vi "Benchmark (SubVI).vi"(10 "Tag Lookup":enum32{"By Name", "By Ref"}(radio)=enum."By Ref", 11 "#Tags":i32=100000) -> (0 "Values":dbl[](array[numeric]), 1 "Read Time":dbl format="%#_g s", 2 "Write Time":dbl format="%#_g s", 3 "Creation Time":dbl format="%#_g s")   [LabVIEW 2018]
doc: "_Test_"
uses:
  Tag/Tag.lvclass/Tag.ctl
  Core/Tag Core.lvclass/Tag Core.ctl
  9bdda2ff-a9dc-4140-9278-b7922a7097c1.vi
  2d795fc3-3ce1-4465-af3b-7f0aa2d422e4.vi
  f807e1ac-a0a3-4e29-b252-0f3a40794f64.vi
  62b6eeaa-51de-4935-a683-d32b75056f49.vi
  45d263af-4112-4fe1-aae2-d3d76b89cb2f.vi
  Tag/Construct.vi
  2d795fc3-3ce1-4465-af3b-7f0aa2d422e4.vi/dad9aa0d-4427-44e9-8a16-aab4251f8442.vi
  2d795fc3-3ce1-4465-af3b-7f0aa2d422e4.vi/85ef243b-a7be-4ddd-aba5-de1810920a44.vi
  f807e1ac-a0a3-4e29-b252-0f3a40794f64.vi/b0e6ee81-700c-4175-ad68-c0a6ecad06c4.vi
  Core/Get Tag.vi
  f807e1ac-a0a3-4e29-b252-0f3a40794f64.vi/af024140-0f6e-4ec8-bc40-cd99cce420e6.vi
  62b6eeaa-51de-4935-a683-d32b75056f49.vi/23fa4edd-30cd-4554-957f-93b0c616928a.vi
  62b6eeaa-51de-4935-a683-d32b75056f49.vi/45e37831-75fa-4a91-aa24-5e089f5f592b.vi
  45d263af-4112-4fe1-aae2-d3d76b89cb2f.vi/a499805a-9911-40c2-9faf-cbd2dbdf1bc0.vi
  45d263af-4112-4fe1-aae2-d3d76b89cb2f.vi/4da4ad56-3947-4053-a029-ec9f142512c4.vi
  Tag/Write Value with Timestamp.vi
  Tag/Read Value.vi
  Tag/Read Timestamp.vi
  Tools/Variant to DBL.vi
  Tag/Set Properties from Initial.vi
  Core/Add Tag.vi
  Core/Get Tag LUT.vi
  <vilib>/Utility/error.llb/Error Cluster From Error Code.vi
  <vilib>/Utility/Data Type/Get Type Information.vi
  Tag/Tag.lvclass
  Core/Tag Core.lvclass
panel:
  out "Read Time / Tag":dbl format="%#_g s"
  out "Write Time / Tag":dbl format="%#_g s"
  out "Creation Time / Tag":dbl format="%#_g s"
  # "Totals"
  # "Per Tag"
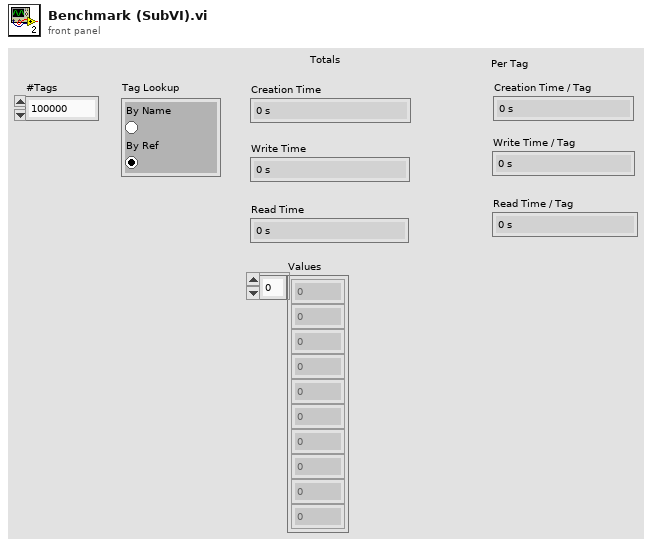
[diagram p1: front panel]
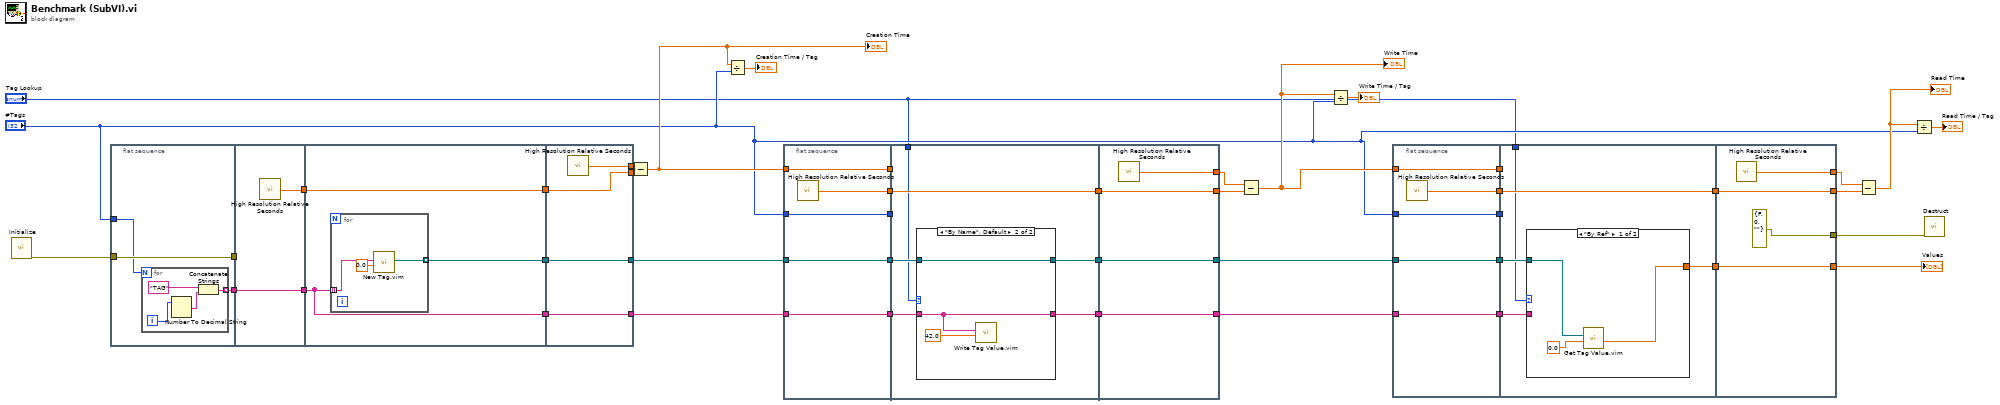
[diagram p0: block diagram]
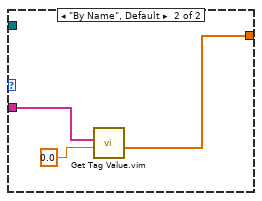
[diagram p2: hidden frame]
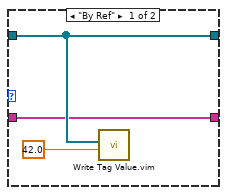
[diagram p3: hidden frame]
diagram:
  n1 = call "Initialize.vi"() -> ("error out"=w39:errorcluster)  [unwired: 11 in]
  n2 = flat-sequence {
    tunnel: w39 -> [w46]
    tunnel: "#Tags" -> [w45]
    tunnel: [w46] -> w23
    tunnel: [w44] -> w21
    tunnel: [w52] -> w42
    tunnel: w23 -> [_]
    tunnel: [w51] -> w22
    tunnel: w21 -> [w51]
    tunnel: [w55] -> w43
    tunnel: w42 -> [w55]
    tunnel: w22 -> [w54]
    tunnel: [w54] -> w18
    tunnel: [w53] -> w7
    tunnel: w43 -> [w61]
    tunnel: [w62] -> w41
    tunnel: [w61] -> w40
    tunnel: [w60] -> w19
    tunnel: w18 -> [w60]
    tunnel: [w59] -> w5
    tunnel: w7 -> [w59]
    frame #0 {
      n3 = for {
        N: w45 -> [_]
        tunnel: [w47] -> w44 mode=indexing
        i -> [w48]
        n4 = Number To Decimal String(number=w48) -> (decimal integer string=w50:string)  [unwired: 1 in]
        n5 = Concatenate Strings("TAG", w50) -> (w47:string)
      }
    }
    frame #1 {
      n6 = call <vilib>:"High Resolution Relative Seconds.vi"() -> ("relative seconds"=w52:dbl)
    }
    frame #2 {
      n7 = for {
        tunnel: w54 -> [w57] mode=indexing
        tunnel: [w56] -> w53 mode=indexing
        n8 = call "New Tag.vim"("Initial Value"=0.0, "Tag Name"=w57) -> ("Tag Ref out"=w56:refnum<data-value>)  [unwired: 8 in, 1 out]
      }
    }
    frame #3 {
      n9 = call <vilib>:"High Resolution Relative Seconds.vi"() -> ("relative seconds"=w62:dbl)
    }
  }
  n10 = Subtract(x=w41, y=w40) -> (x-y=w14:dbl)
  "Creation Time" <- w14
  n11 = Divide(x=w14, y="#Tags") -> (x/y=→"Creation Time / Tag":dbl)
  n12 = flat-sequence {
    tunnel: w14 -> [w67]
    tunnel: [w67] -> w38
    tunnel: [w66] -> w36
    tunnel: [w65] -> w35
    tunnel: "#Tags" -> [w65]
    tunnel: [w64] -> w20
    tunnel: w19 -> [w64]
    tunnel: [w63] -> w6
    tunnel: w5 -> [w63]
    tunnel: w38 -> [_]
    tunnel: [w73] -> w37
    tunnel: w36 -> [w73]
    tunnel: w35 -> [_]
    tunnel: w20 -> [w70]
    tunnel: [w69] -> w15
    tunnel: w6 -> [w72]
    tunnel: [w68] -> w2
    tunnel: "Tag Lookup" -> [w71]
    tunnel: w37 -> [w83]
    tunnel: [w83] -> w33
    tunnel: [w82] -> w34
    tunnel: [w81] -> w16
    tunnel: w15 -> [w81]
    tunnel: [w80] -> w3
    tunnel: w2 -> [w80]
    frame #0 {
      n13 = call <vilib>:"High Resolution Relative Seconds.vi"() -> ("relative seconds"=w66:dbl)
    }
    frame #1 {
      n14 = case shown="\"By Name\", Default" w71 {
        tunnel: w72 -> [w75 w77]
        tunnel: w70 -> [w74 w78]
        tunnel: [w74 w78] -> w69
        tunnel: [w75 w77] -> w68
        frame "By Ref" {
          n15 = call "Write Tag Value.vim"("Value"=42.0, "Tag Name(s)/Ref(s)"=w75) -> ()  [unwired: 8 in, 2 out]
        }
        frame "By Name", Default {
          n16 = call "Write Tag Value.vim"("Value"=42.0, "Tag Name(s)/Ref(s)"=w78) -> ()  [unwired: 8 in, 2 out]
        }
      }
    }
    frame #2 {
      n17 = call <vilib>:"High Resolution Relative Seconds.vi"() -> ("relative seconds"=w82:dbl)
    }
  }
  n18 = Subtract(x=w34, y=w33) -> (x-y=w12:dbl)
  "Write Time" <- w12
  n19 = Divide(x=w12, y="#Tags") -> (x/y=→"Write Time / Tag":dbl)
  n20 = flat-sequence {
    tunnel: w12 -> [w88]
    tunnel: [w88] -> w32
    tunnel: [w87] -> w31
    tunnel: [w86] -> w30
    tunnel: "#Tags" -> [w86]
    tunnel: [w85] -> w17
    tunnel: w16 -> [w85]
    tunnel: [w84] -> w4
    tunnel: w3 -> [w84]
    tunnel: w32 -> [_]
    tunnel: [w93] -> w29
    tunnel: w31 -> [w93]
    tunnel: w30 -> [_]
    tunnel: [w92] -> w26
    tunnel: w17 -> [w89]
    tunnel: w4 -> [w91]
    tunnel: "Tag Lookup" -> [w90]
    tunnel: w29 -> [w103]
    tunnel: [w103] -> w28
    tunnel: [w102] -> w27
    tunnel: [w101] -> w25
    tunnel: w26 -> [w101]
    tunnel: [errorcluster {"status"=FALSE, "code"=0, "source"=""} ("error in (no error)")] -> w24
    frame #0 {
      n21 = call <vilib>:"High Resolution Relative Seconds.vi"() -> ("relative seconds"=w87:dbl)
    }
    frame #1 {
      n22 = case shown="\"By Ref\"" w90 {
        tunnel: [w95 w98] -> w92
        tunnel: w91 -> [w94 _]
        tunnel: w89 -> [_ w97]
        frame "By Ref" {
          n23 = call "Get Tag Value.vim"("Default (Void)"=0.0, "Tag Name(s)/Ref(s)"=w94) -> ("Value"=w95:dbl[])  [unwired: 6 in, 3 out]
        }
        frame "By Name", Default {
          n24 = call "Get Tag Value.vim"("Default (Void)"=0.0, "Tag Name(s)/Ref(s)"=w97) -> ("Value"=w98:dbl[])  [unwired: 6 in, 3 out]
        }
      }
    }
    frame #2 {
      n25 = call <vilib>:"High Resolution Relative Seconds.vi"() -> ("relative seconds"=w102:dbl)
    }
  }
  n26 = Subtract(x=w27, y=w28) -> (x-y=w9:dbl)
  "Read Time" <- w9
  n27 = Divide(x=w9, y="#Tags") -> (x/y=→"Read Time / Tag":dbl)
  n28 = call "Destruct.vi"("error in (no error)"=w24) -> ()  [unwired: 10 in, 1 out]
  "Values" <- w25
